vi "Determine Warning 3-8 .vi"() -> ()   [LabVIEW 2014]
panel:
  in  "Minimum Tempature":dbl
  in  "Maximum Tempature":dbl
  in  "Current Temp":dbl
  out "Warning Text":string
  out "Warning":bool
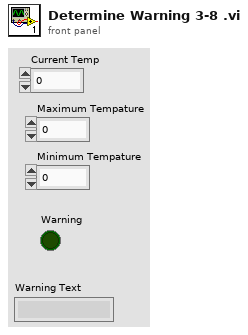
[diagram p1: front panel]
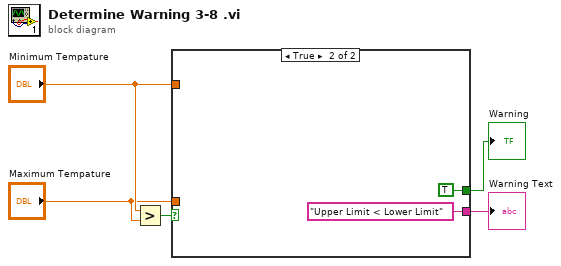
[diagram p0: block diagram]
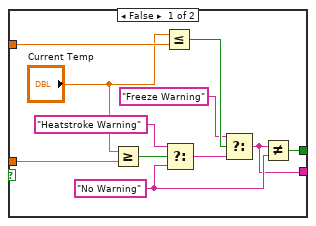
[diagram p2: hidden frame]
diagram:
  n1 = Greater?(x="Minimum Tempature", y="Maximum Tempature") -> (0:w1:bool)
  n2 = case shown="True" w1 {
    tunnel: "Minimum Tempature" -> [w16 _]
    tunnel: "Maximum Tempature" -> [w15 _]
    tunnel: [w7 TRUE] -> w5
    tunnel: [w6 "Upper Limit < Lower Limit"] -> w4
    frame False {
      w11 = "No Warning"
      n3 = Greater Or Equal?(x="Current Temp", y=w15) -> (x >= y?=w13:bool)
      n4 = Less Or Equal?(x="Current Temp", y=w16) -> (x <= y?=w10:bool)
      n5 = Select(t="Heatstroke Warning", s=w13, f=w11) -> (s? t:f=w8:string)
      n6 = Select(t="Freeze Warning", s=w10, f=w8) -> (s? t:f=w6:string)
      n7 = Not Equal?(x=w6, y=w11) -> (x != y?=w7:bool)
    }
    frame True {
    }
  }
  "Warning" <- w5
  "Warning Text" <- w4
